vi "Go.vi"(9 "Timing Data":T1(array[cluster]), 10 "Control In":T2={"I-O.lvclass"=refnum, "Gantry"=refnum, "Dispenser"="COM1"}, 11 "Sensor Dispense in":refnum<class "Sensor Dispense.lvclass">) -> (2 "Control Out":T2={"I-O.lvclass"=refnum, "Gantry"=refnum, "Dispenser"="COM1"}, 3 "Sensor Dispense out":refnum<class "Sensor Dispense.lvclass">)   [LabVIEW 2018, in "Sensor Dispense.lvclass"]
uses:
  Sensor Dispense.lvclass
  C:/Users/HEP/Documents/GitHub/New folder/C/Users/HEP/Documents/GitHub/UCSB-Gantry-HEP-2018/Classes/Routine/Dispense/Dispense.lvclass
  Classes/Controller/Controllers.ctl
  Classes/Controller/I-O/I-O.lvclass
  C:/Program Files (x86)/Aerotech/A3200/LabVIEW/2010/Bin/Aerotech.A3200.dll
  Program Files (x86)/Aerotech/A3200/LabVIEW/2010/Bin/Aerotech.A3200.dll
  Sensor Dispense.lvclass/Sensor Dispense.ctl
  Classes/Controller/Motion/Motion.lvclass
  Classes/Controller/Dispenser/Dispenser.lvclass
  Classes/Controller/Motion/A3200/A3200.lvclass
  Classes/Controller/Controller.lvclass
panel:
  out "error out":errorcluster
  in  "error in (no error)":errorcluster
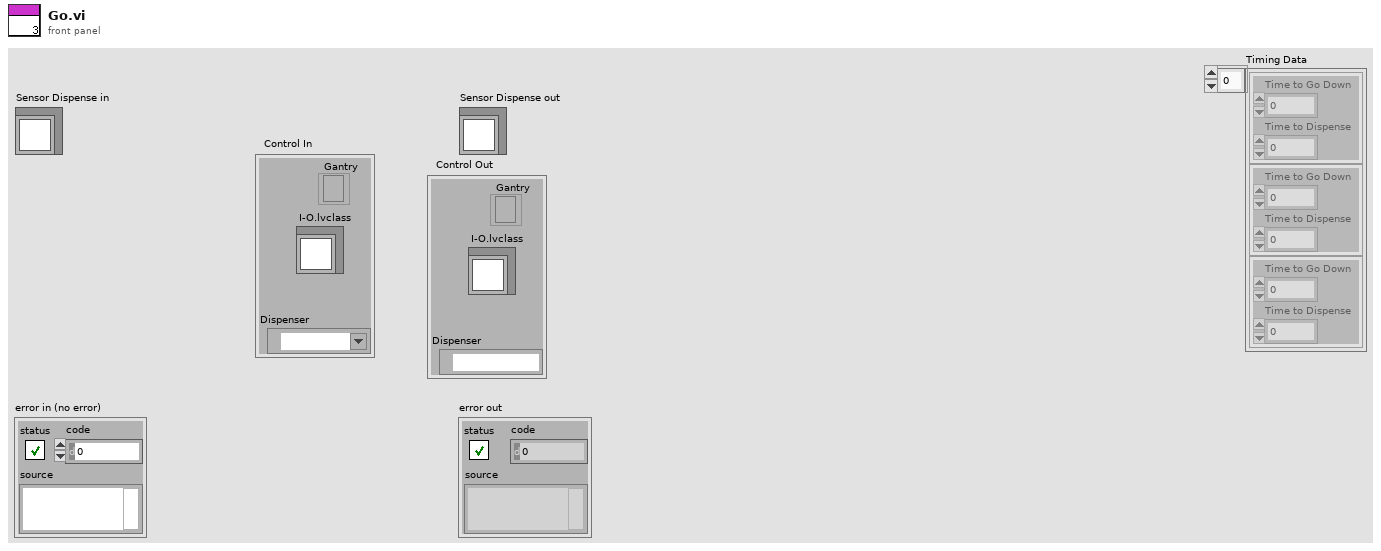
[diagram p1: front panel]
types:
  T1 = cluster{"Time to Go Down":i32, "Time to Dispense":i32}[]
  T2 = typedef "Controller.lvclass/Controllers.ctl" = cluster{"I-O.lvclass":refnum<class "I-O.lvclass">, "Gantry":refnum<k24>, "Dispenser":refnum<visa-resource-name>}
  T3 = cluster{"Endpoints":dbl[][], "Center":dbl[], "CW/CCW":dbl, "Dispense Type":enum16{"N-gon", "Square", "Arc", "Dot", "Line", "Circle"}}[]
  T4 = enum16{"N-gon", "Square", "Arc", "Dot", "Line", "Circle"}
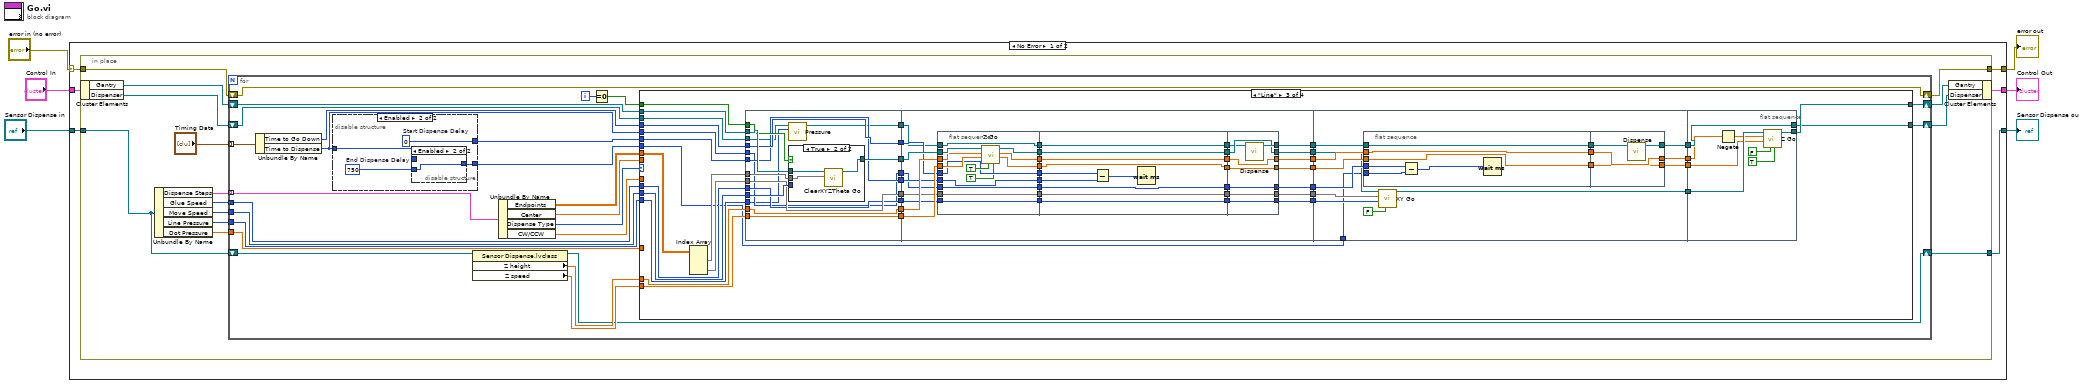
[diagram p0: block diagram]
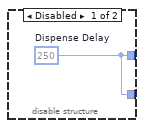
[diagram p2: hidden frame]
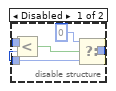
[diagram p3: hidden frame]
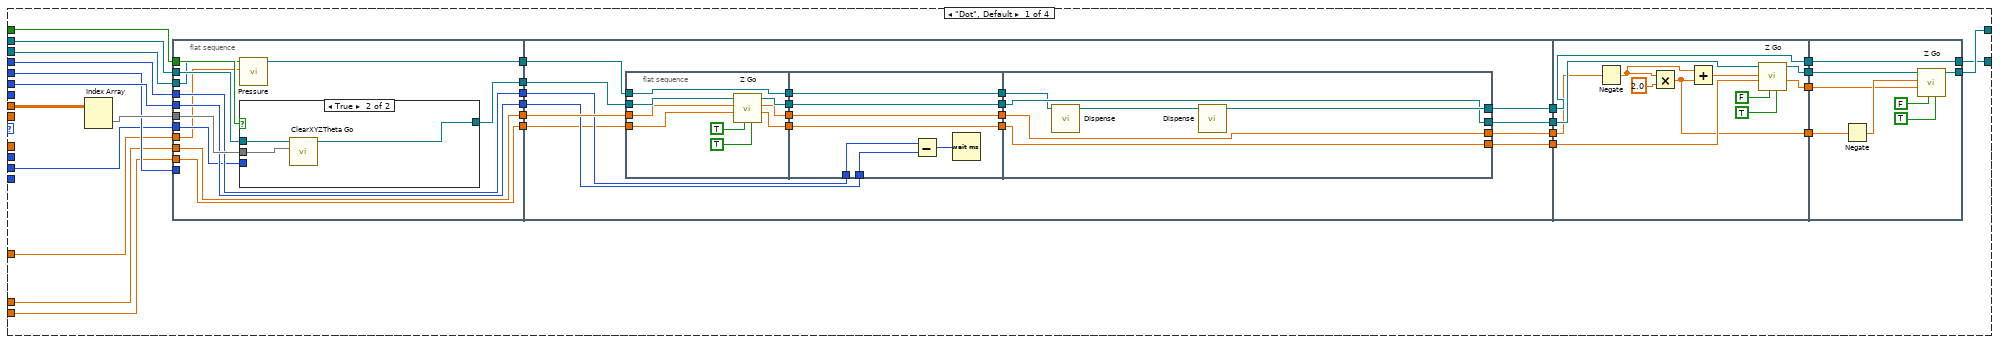
[diagram p4: hidden frame]
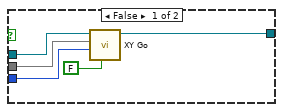
[diagram p5: hidden frame]
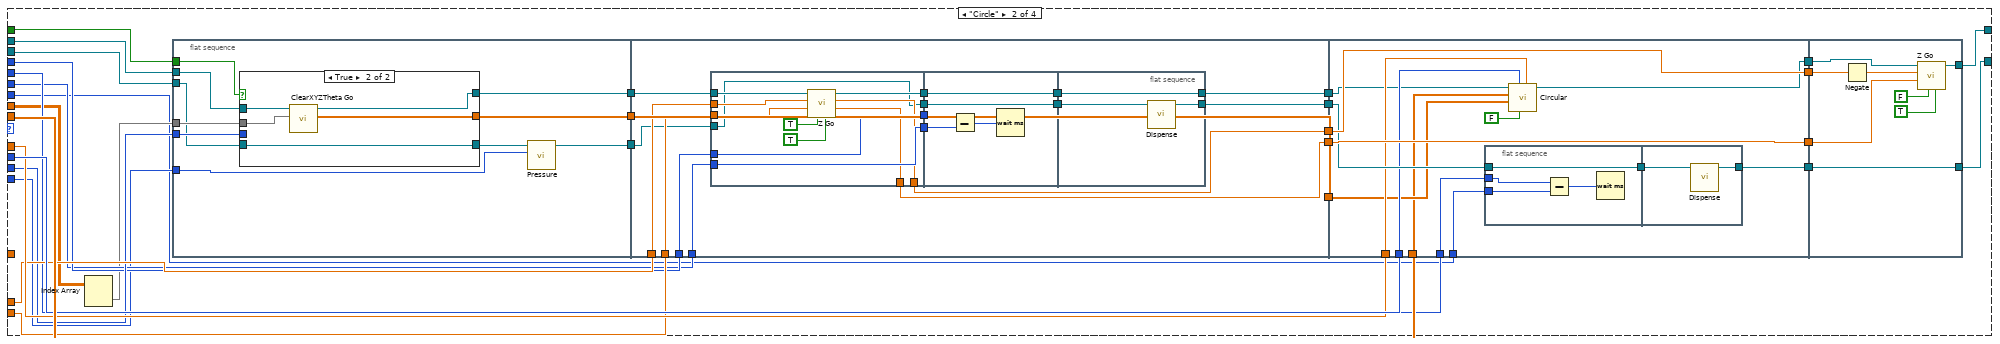
[diagram p6: hidden frame]
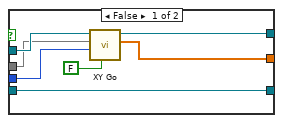
[diagram p7: hidden frame]
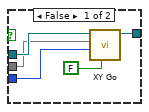
[diagram p8: hidden frame]
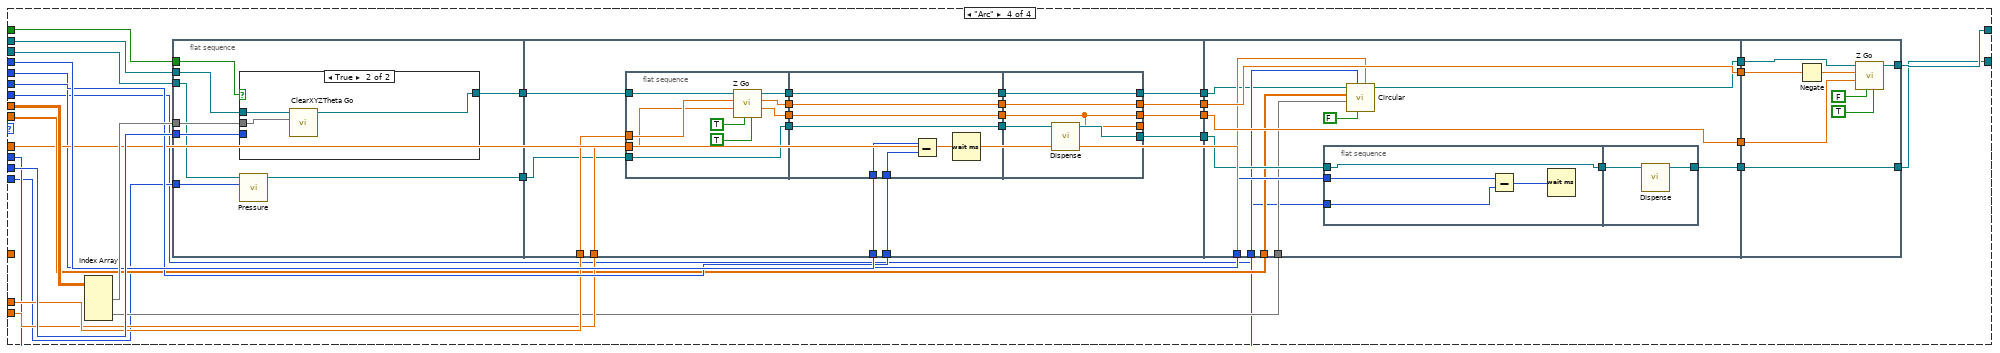
[diagram p9: hidden frame]
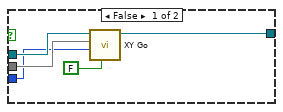
[diagram p10: hidden frame]
diagram:
  n1 = case shown="No Error" "error in (no error)" {
    selector: "error in (no error)" -> [w7 w559]
    tunnel: "Sensor Dispense in" -> [w12 w558]
    tunnel: [w11 w558] -> w5
    tunnel: "Control In" -> [w10 w557]
    tunnel: [w9 w557] -> w3
    tunnel: [w8 w559] -> w2
    frame No Error {
      n2 = in-place {
        in-place-border: w12 -> [w24]
        in-place-border: [w23] -> w11
        in-place-border: w7 -> [w17]
        in-place-border: [w16] -> w8
        n3 = in-place-cluster #1(w10) -> ("Gantry"=w25:refnum<k24>, "Dispenser"=w20:refnum<visa-resource-name>)
        n4 = Unbundle By Name(w24) -> ("Dispense Steps"=w21:T3, "Glue Speed"=w15:i32, "Move Speed"=w26:i32, "Line Pressure"=w13:i64, "Dot Pressure"=w14:dbl)
        n5 = for {
          tunnel: w26 -> [w51]
          shift-right: [w42] -> w22
          shift-left: w25 -> [w49]
          tunnel: w15 -> [w50]
          shift-right: [w34] -> w23
          shift-left: w24 -> [w47]
          tunnel: w21 -> [w44] mode=indexing
          shift-right: [w37] -> w18
          shift-left: w20 -> [w40]
          tunnel: "Timing Data" -> [w39] mode=indexing
          shift-right: [w29] -> w16
          shift-left: w17 -> [w29]
          tunnel: w14 -> [w31]
          tunnel: w13 -> [w30]
          i -> [w46]
          n6 = Unbundle By Name(w39) -> ("Time to Go Down"=w38:i32, "Time to Dispense"=w27:i32)
          n7 = disable-structure shown="Enabled" {
            disable-tunnel: [w52 w56] -> w33
            disable-tunnel: [w52 w54] -> w28
            disable-tunnel: w27 -> [_ w55]
            frame Disabled {
              w52 = 250  # Dispense Delay
            }
            frame Enabled {
              w53 = 750  # End Dispense Delay
              w56 = 0  # Start Dispense Delay
              n8 = disable-structure shown="Enabled" {
                disable-tunnel: w55 -> [w61 _]
                disable-tunnel: [w58 w62] -> w54
                disable-tunnel: w53 -> [w57 w62]
                frame Disabled {
                  n9 = Less?(x=w61, y=w57) -> (x < y?=w60:bool)
                  n10 = Select(t=0, s=w60, f=w57) -> (s? t:f=w58:i32)
                }
                frame Enabled {
                }
              }
            }
          }
          n11 = property class="Sensor Dispense.lvclass"(reference=w47) -> (reference out=w34:refnum<class "Sensor Dispense.lvclass">, "Z height"=w36:dbl, "Z speed"=w35:dbl)  [unwired: 1 in, 1 out]
          n12 = Unbundle By Name(w44) -> ("Endpoints"=w32:dbl[][], "Center"=w41:dbl[], "Dispense Type"=w43:T4, "CW/CCW"=w48:dbl)
          n13 = Equal To 0?(x=w46) -> (x = 0?=w45:bool)
          n14 = case shown="\"Line\"" w43 {
            tunnel: w41 -> [_ w196 _ w455]
            tunnel: w49 -> [w89 w197 w323 w464]
            tunnel: w51 -> [w72 w190 w322 w461]
            tunnel: [w88 w200 w319 w451] -> w42
            tunnel: w50 -> [_ w195 w309 w454]
            tunnel: w48 -> [_ w194 _ w453]
            tunnel: w35 -> [w80 w192 w306 w457]
            tunnel: w36 -> [w81 w193 w307 w458]
            tunnel: w45 -> [w90 w191 w321 w465]
            tunnel: w40 -> [w79 w174 w313 w447]
            tunnel: w38 -> [w77 w181 w311 w460]
            tunnel: w27 -> [w82 w182 w308 w452]
            tunnel: w33 -> [w83 w180 w312 w459]
            tunnel: [w87 w175 w316 w450] -> w37
            tunnel: w32 -> [w86 w179 w315 w463]
            tunnel: w31 -> [w71 _ _ _]
            tunnel: w30 -> [_ w172 w288 w446]
            tunnel: w28 -> [_ w171 w287 w445]
            frame "Dot", Default {
              n15 = Index Array(array=w86) -> (element=w85:dbl[])  [unwired: 2 in]
              n16 = flat-sequence {
                tunnel: w90 -> [w102]
                tunnel: w89 -> [w101]
                tunnel: w85 -> [w100]
                tunnel: [w99] -> w84
                tunnel: w83 -> [w96]
                tunnel: w82 -> [_]
                tunnel: w81 -> [w98]
                tunnel: w80 -> [w95]
                tunnel: w79 -> [w93]
                tunnel: [w98] -> w78
                tunnel: w77 -> [w97]
                tunnel: [w97] -> w76
                tunnel: [w96] -> w75
                tunnel: [w92] -> w74
                tunnel: [w95] -> w73
                tunnel: w72 -> [w94]
                tunnel: w71 -> [w91]
                tunnel: [w128] -> w68
                tunnel: w84 -> [w127]
                tunnel: [w124] -> w67
                tunnel: w78 -> [w123]
                tunnel: w76 -> [w122]
                tunnel: w75 -> [w121]
                tunnel: w74 -> [w120]
                tunnel: w73 -> [w117]
                tunnel: [w114] -> w66
                tunnel: [w113] -> w65
                tunnel: w68 -> [w161]
                tunnel: w67 -> [w160]
                tunnel: w66 -> [w159]
                tunnel: w65 -> [w156]
                tunnel: [w162] -> w70
                tunnel: [w161] -> w69
                tunnel: [w155] -> w64
                tunnel: [w151] -> w63
                tunnel: [w170] -> w87
                tunnel: [w168] -> w88
                tunnel: w70 -> [w169]
                tunnel: w69 -> [w170]
                tunnel: w64 -> [w166]
                tunnel: w63 -> [w163]
                frame #0 {
                  n17 = call "Pressure.vi"("Pressure"=w91, "VISA resource name"=w93) -> ("VISA resource name out"=w92:refnum<visa-resource-name>)  [unwired: 8 in, 1 out]
                  n18 = case shown="True" w102 {
                    tunnel: w101 -> [w107 w110]
                    tunnel: [w106 w109] -> w99
                    tunnel: w100 -> [w105 w108]
                    tunnel: w94 -> [w104 _]
                    frame False {
                      n19 = call "XY Go.vi"("return immediately"=FALSE, "Speed"=w104, "XY In"=w105, "Gantry In"=w107) -> ("Gantry Out"=w106:refnum<k24>)  [unwired: 5 in, 2 out]
                    }
                    frame True {
                      n20 = call "ClearXYZTheta Go.vi"("XYZTheta In"=w108, "Gantry In"=w110) -> ("Gantry Out"=w109:refnum<k24>)  [unwired: 7 in, 2 out]
                    }
                  }
                }
                frame #1 {
                  n21 = flat-sequence {
                    tunnel: w127 -> [w137]
                    tunnel: [w136] -> w125
                    tunnel: w123 -> [w129]
                    tunnel: w120 -> [w134]
                    tunnel: [w134] -> w119
                    tunnel: w117 -> [w133]
                    tunnel: [w132] -> w116
                    tunnel: [w131] -> w111
                    tunnel: [w144] -> w126
                    tunnel: w125 -> [w144]
                    tunnel: w122 -> [w143]
                    tunnel: w121 -> [w139]
                    tunnel: w119 -> [w142]
                    tunnel: [w142] -> w118
                    tunnel: w116 -> [w141]
                    tunnel: [w141] -> w115
                    tunnel: [w140] -> w112
                    tunnel: w111 -> [w140]
                    tunnel: [w150] -> w128
                    tunnel: w126 -> [w149]
                    tunnel: [w149] -> w124
                    tunnel: w118 -> [w148]
                    tunnel: w115 -> [w146]
                    tunnel: [w146] -> w114
                    tunnel: [w145] -> w113
                    tunnel: w112 -> [w145]
                    frame #0 {
                      n22 = call "Z Go.vi"("Increment"=TRUE, "Return Immediately"=TRUE, "Speed In"=w133, "Position In"=w129, "Gantry In"=w137) -> ("Speed Out"=w131:dbl, "Position Out"=w132:dbl, "Gantry Out"=w136:refnum<k24>)  [unwired: 3 in, 1 out]
                    }
                    frame #1 {
                      n23 = Subtract(x=w143, y=w139) -> (x-y=w138:i32)
                      n24 = Wait (ms)(milliseconds to wait=w138) -> ()  [unwired: 1 out]
                    }
                    frame #2 {
                      n25 = call "Dispense.vi"("Dispenser In"=w148) -> ("Dispenser Out"=w147:refnum<visa-resource-name>)  [unwired: 9 in, 1 out]
                      n26 = call "Dispense.vi"("Dispenser In"=w147) -> ("Dispenser Out"=w150:refnum<visa-resource-name>)  [unwired: 9 in, 1 out]
                    }
                  }
                }
                frame #2 {
                  n27 = Negate(x=w159) -> (-x=w153:dbl)
                  n28 = Multiply(x=w153, y=2.0) -> (x*y=w151:dbl)
                  n29 = Add(x=w153, y=w151) -> (x+y=w154:dbl)
                  n30 = call "Z Go.vi"("Increment"=TRUE, "Return Immediately"=FALSE, "Speed In"=w156, "Position In"=w154, "Gantry In"=w160) -> ("Speed Out"=w155:dbl, "Gantry Out"=w162:refnum<k24>)  [unwired: 3 in, 2 out]
                }
                frame #3 {
                  n31 = Negate(x=w163) -> (-x=w167:dbl)
                  n32 = call "Z Go.vi"("Increment"=TRUE, "Return Immediately"=FALSE, "Speed In"=w166, "Position In"=w167, "Gantry In"=w169) -> ("Gantry Out"=w168:refnum<k24>)  [unwired: 3 in, 3 out]
                }
              }
            }
            frame "Circle" {
              n33 = Index Array(array=w179) -> (element=w178:dbl[])  [unwired: 2 in]
              n34 = flat-sequence {
                tunnel: [w208] -> w199
                tunnel: w197 -> [w209]
                tunnel: w191 -> [w210]
                tunnel: w190 -> [w207]
                tunnel: [w206] -> w188
                tunnel: w178 -> [w205]
                tunnel: w174 -> [w204]
                tunnel: [w202] -> w173
                tunnel: w172 -> [w201]
                tunnel: w193 -> [w232]
                tunnel: w192 -> [w233]
                tunnel: [w239] -> w189
                tunnel: [w230] -> w187
                tunnel: [w231] -> w186
                tunnel: w188 -> [w239]
                tunnel: w199 -> [w229]
                tunnel: [w238] -> w183
                tunnel: w181 -> [w237]
                tunnel: w180 -> [w236]
                tunnel: [w226] -> w177
                tunnel: w173 -> [w225]
                tunnel: [w260] -> w198
                tunnel: [w272] -> w185
                tunnel: [w271] -> w184
                tunnel: w182 -> [w270]
                tunnel: w183 -> [w268]
                tunnel: w189 -> [w263]
                tunnel: w187 -> [w272]
                tunnel: w186 -> [w271]
                tunnel: w194 -> [w266]
                tunnel: w195 -> [w264]
                tunnel: w196 -> [w262]
                tunnel: w177 -> [w261]
                tunnel: [w269] -> w176
                tunnel: w171 -> [w259]
                tunnel: [w284] -> w200
                tunnel: w198 -> [w285]
                tunnel: w185 -> [w286]
                tunnel: w184 -> [w283]
                tunnel: w176 -> [w282]
                tunnel: [w282] -> w175
                frame #0 {
                  n35 = case shown="True" w210 {
                    tunnel: w209 -> [w217 w222]
                    tunnel: [w216 w221] -> w208
                    tunnel: w207 -> [w215 _]
                    tunnel: [w214 w219] -> w206
                    tunnel: w205 -> [w213 w220]
                    tunnel: w204 -> [w212 w218]
                    tunnel: [w212 w218] -> w203
                    frame False {
                      n36 = call "XY Go.vi"("return immediately"=FALSE, "Speed"=w215, "XY In"=w213, "Gantry In"=w217) -> ("XY Out"=w214:dbl[], "Gantry Out"=w216:refnum<k24>)  [unwired: 5 in, 1 out]
                    }
                    frame True {
                      n37 = call "ClearXYZTheta Go.vi"("XYZTheta In"=w220, "Gantry In"=w222) -> ("XYZTheta Out"=w219:dbl[], "Gantry Out"=w221:refnum<k24>)  [unwired: 7 in, 1 out]
                    }
                  }
                  n38 = call "Pressure.vi"("Pressure"=w201, "VISA resource name"=w203) -> ("VISA resource name out"=w202:refnum<visa-resource-name>)  [unwired: 8 in, 1 out]
                }
                frame #1 {
                  n39 = flat-sequence {
                    tunnel: w236 -> [w249]
                    tunnel: w237 -> [w250]
                    tunnel: [w250] -> w235
                    tunnel: [w249] -> w234
                    tunnel: w233 -> [w248]
                    tunnel: w232 -> [w247]
                    tunnel: [w246] -> w231
                    tunnel: [w245] -> w230
                    tunnel: w229 -> [w244]
                    tunnel: [w243] -> w228
                    tunnel: w225 -> [w241]
                    tunnel: [w241] -> w224
                    tunnel: w235 -> [w255]
                    tunnel: w234 -> [w254]
                    tunnel: w228 -> [w253]
                    tunnel: [w253] -> w227
                    tunnel: w224 -> [w252]
                    tunnel: [w252] -> w223
                    tunnel: [w258] -> w238
                    tunnel: w227 -> [w257]
                    tunnel: [w257] -> w226
                    tunnel: w223 -> [w256]
                    frame #0 {
                      n40 = call "Z Go.vi"("Increment"=TRUE, "Return Immediately"=TRUE ("return immediately"), "Speed In"=w248, "Position In"=w247, "Gantry In"=w244) -> ("Speed Out"=w246:dbl, "Position Out"=w245:dbl, "Gantry Out"=w243:refnum<k24>)  [unwired: 3 in, 1 out]
                    }
                    frame #1 {
                      n41 = Subtract(x=w255, y=w254) -> (x-y=w251:i32)
                      n42 = Wait (ms)(milliseconds to wait=w251) -> ()  [unwired: 1 out]
                    }
                    frame #2 {
                      n43 = call "Dispense.vi"("Dispenser In"=w256) -> ("Dispenser Out"=w258:refnum<visa-resource-name>)  [unwired: 9 in, 1 out]
                    }
                  }
                }
                frame #2 {
                  n44 = flat-sequence {
                    tunnel: [w274] -> w267
                    tunnel: w270 -> [w276]
                    tunnel: w268 -> [w274]
                    tunnel: w259 -> [w273]
                    tunnel: [w278] -> w269
                    tunnel: w267 -> [w277]
                    frame #0 {
                      n45 = Subtract(x=w276, y=w273) -> (x-y=w275:i32)
                      n46 = Wait (ms)(milliseconds to wait=w275) -> ()  [unwired: 1 out]
                    }
                    frame #1 {
                      n47 = call "Dispense.vi"("Dispenser In"=w277) -> ("Dispenser Out"=w278:refnum<visa-resource-name>)  [unwired: 9 in, 1 out]
                    }
                  }
                  n48 = call "Circular.vi"("Direction"=w266, "return immediately"=FALSE, "Speed"=w264, "XY End"=w263, "XY Center"=w262, "Gantry In"=w261) -> ("Gantry Out"=w260:refnum<k24>)  [unwired: 4 in, 1 out]
                }
                frame #3 {
                  n49 = Negate(x=w286) -> (-x=w281:dbl)
                  n50 = call "Z Go.vi"("Increment"=TRUE, "Return Immediately"=FALSE, "Speed In"=w283, "Position In"=w281, "Gantry In"=w285) -> ("Gantry Out"=w284:refnum<k24>)  [unwired: 3 in, 3 out]
                }
              }
            }
            frame "Line" {
              n51 = Index Array(array=w315) -> (element #1=w314:dbl[], element #2=w310:dbl[])  [unwired: 4 in]
              n52 = flat-sequence {
                tunnel: w323 -> [w338]
                tunnel: w322 -> [w337]
                tunnel: w321 -> [w336]
                tunnel: [w335] -> w320
                tunnel: w314 -> [w334]
                tunnel: w313 -> [w326]
                tunnel: w312 -> [w330]
                tunnel: w311 -> [w331]
                tunnel: w310 -> [w329]
                tunnel: w309 -> [w328]
                tunnel: w308 -> [w327]
                tunnel: w307 -> [w333]
                tunnel: w306 -> [w332]
                tunnel: [w333] -> w305
                tunnel: [w332] -> w304
                tunnel: [w331] -> w302
                tunnel: [w330] -> w301
                tunnel: [w325] -> w300
                tunnel: [w329] -> w298
                tunnel: [w328] -> w296
                tunnel: [w327] -> w294
                tunnel: w288 -> [w324]
                tunnel: w320 -> [w377]
                tunnel: [w378] -> w318
                tunnel: w305 -> [w376]
                tunnel: w304 -> [w375]
                tunnel: [w372] -> w303
                tunnel: w302 -> [w370]
                tunnel: w301 -> [w368]
                tunnel: w300 -> [w365]
                tunnel: [w364] -> w299
                tunnel: w298 -> [w361]
                tunnel: [w360] -> w297
                tunnel: w296 -> [w357]
                tunnel: [w353] -> w295
                tunnel: w294 -> [w354]
                tunnel: [w352] -> w291
                tunnel: [w349] -> w289
                tunnel: w318 -> [w424]
                tunnel: [w426] -> w317
                tunnel: w303 -> [w413]
                tunnel: w299 -> [w414]
                tunnel: w297 -> [w415]
                tunnel: w295 -> [w423]
                tunnel: [w412] -> w293
                tunnel: [w422] -> w292
                tunnel: w291 -> [w420]
                tunnel: [w419] -> w290
                tunnel: w289 -> [w417]
                tunnel: w287 -> [w411]
                tunnel: [w444] -> w319
                tunnel: w317 -> [w443]
                tunnel: [w443] -> w316
                tunnel: w293 -> [w442]
                tunnel: w292 -> [w441]
                tunnel: w290 -> [w439]
                frame #0 {
                  n53 = call "Pressure.vi"("Pressure"=w324, "VISA resource name"=w326) -> ("VISA resource name out"=w325:refnum<visa-resource-name>)  [unwired: 8 in, 1 out]
                  n54 = case shown="True" w336 {
                    tunnel: w338 -> [w343 w346]
                    tunnel: w337 -> [w342 _]
                    tunnel: [w341 w345] -> w335
                    tunnel: w334 -> [w340 w344]
                    frame False {
                      n55 = call "XY Go.vi"("return immediately"=FALSE, "Speed"=w342, "XY In"=w340, "Gantry In"=w343) -> ("Gantry Out"=w341:refnum<k24>)  [unwired: 5 in, 2 out]
                    }
                    frame True {
                      n56 = call "ClearXYZTheta Go.vi"("XYZTheta In"=w344, "Gantry In"=w346) -> ("Gantry Out"=w345:refnum<k24>)  [unwired: 7 in, 2 out]
                    }
                  }
                }
                frame #1 {
                  n57 = flat-sequence {
                    tunnel: w377 -> [w392]
                    tunnel: w376 -> [w391]
                    tunnel: w375 -> [w390]
                    tunnel: [w388] -> w374
                    tunnel: [w387] -> w371
                    tunnel: w370 -> [w387]
                    tunnel: [w386] -> w369
                    tunnel: w368 -> [w386]
                    tunnel: [w385] -> w366
                    tunnel: w365 -> [w385]
                    tunnel: [w384] -> w362
                    tunnel: w361 -> [w384]
                    tunnel: [w383] -> w358
                    tunnel: w357 -> [w383]
                    tunnel: [w382] -> w355
                    tunnel: w354 -> [w382]
                    tunnel: [w381] -> w350
                    tunnel: [w380] -> w347
                    tunnel: w374 -> [w402]
                    tunnel: [w402] -> w373
                    tunnel: w371 -> [w401]
                    tunnel: w369 -> [w396]
                    tunnel: [w400] -> w367
                    tunnel: w366 -> [w400]
                    tunnel: [w399] -> w363
                    tunnel: w362 -> [w399]
                    tunnel: [w398] -> w359
                    tunnel: w358 -> [w398]
                    tunnel: [w397] -> w356
                    tunnel: w355 -> [w397]
                    tunnel: [w395] -> w351
                    tunnel: w350 -> [w395]
                    tunnel: [w394] -> w348
                    tunnel: w347 -> [w394]
                    tunnel: [w410] -> w378
                    tunnel: w373 -> [w409]
                    tunnel: [w409] -> w372
                    tunnel: w367 -> [w405]
                    tunnel: [w408] -> w364
                    tunnel: w363 -> [w408]
                    tunnel: [w407] -> w360
                    tunnel: w359 -> [w407]
                    tunnel: w356 -> [w406]
                    tunnel: [w406] -> w353
                    tunnel: [w404] -> w352
                    tunnel: w351 -> [w404]
                    tunnel: [w403] -> w349
                    tunnel: w348 -> [w403]
                    frame #0 {
                      n58 = call "Z Go.vi"("Increment"=TRUE, "Return Immediately"=TRUE, "Speed In"=w390, "Position In"=w391, "Gantry In"=w392) -> ("Speed Out"=w380:dbl, "Position Out"=w381:dbl, "Gantry Out"=w388:refnum<k24>)  [unwired: 3 in, 1 out]
                    }
                    frame #1 {
                      n59 = Subtract(x=w401, y=w396) -> (x-y=w393:i32)
                      n60 = Wait (ms)(milliseconds to wait=w393) -> ()  [unwired: 1 out]
                    }
                    frame #2 {
                      n61 = call "Dispense.vi"("Dispenser In"=w405) -> ("Dispenser Out"=w410:refnum<visa-resource-name>)  [unwired: 9 in, 1 out]
                    }
                  }
                }
                frame #2 {
                  n62 = flat-sequence {
                    tunnel: [w432] -> w425
                    tunnel: [w430] -> w421
                    tunnel: [w429] -> w418
                    tunnel: w424 -> [w432]
                    tunnel: w423 -> [w431]
                    tunnel: w420 -> [w430]
                    tunnel: w417 -> [w429]
                    tunnel: w411 -> [w427]
                    tunnel: [w436] -> w426
                    tunnel: w425 -> [w435]
                    tunnel: [w434] -> w422
                    tunnel: w421 -> [w434]
                    tunnel: [w433] -> w419
                    tunnel: w418 -> [w433]
                    frame #0 {
                      n63 = Subtract(x=w431, y=w427) -> (x-y=w428:i32)
                      n64 = Wait (ms)(milliseconds to wait=w428) -> ()  [unwired: 1 out]
                    }
                    frame #1 {
                      n65 = call "Dispense.vi"("Dispenser In"=w435) -> ("Dispenser Out"=w436:refnum<visa-resource-name>)  [unwired: 9 in, 1 out]
                    }
                  }
                  n66 = call "XY Go.vi"("return immediately"=FALSE, "Speed"=w415, "XY In"=w414, "Gantry In"=w413) -> ("Gantry Out"=w412:refnum<k24>)  [unwired: 5 in, 2 out]
                }
                frame #3 {
                  n67 = Negate(x=w441) -> (-x=w440:dbl)
                  n68 = call "Z Go.vi"("Increment"=TRUE, "Return Immediately"=FALSE, "Speed In"=w439, "Position In"=w440, "Gantry In"=w442) -> ("Gantry Out"=w444:refnum<k24>)  [unwired: 3 in, 3 out]
                }
              }
            }
            frame "Arc" {
              n69 = Index Array(array=w463) -> (element #1=w462:dbl[], element #2=w456:dbl[])  [unwired: 4 in]
              n70 = flat-sequence {
                tunnel: [w481] -> w473
                tunnel: w465 -> [w480]
                tunnel: w464 -> [w479]
                tunnel: w462 -> [w478]
                tunnel: w461 -> [w477]
                tunnel: [w476] -> w448
                tunnel: w447 -> [w475]
                tunnel: w446 -> [w474]
                tunnel: w473 -> [w506]
                tunnel: [w507] -> w472
                tunnel: [w503] -> w471
                tunnel: [w500] -> w470
                tunnel: [w497] -> w469
                tunnel: w460 -> [w496]
                tunnel: w459 -> [w495]
                tunnel: w458 -> [w494]
                tunnel: w457 -> [w493]
                tunnel: w448 -> [w492]
                tunnel: w472 -> [w538]
                tunnel: [w539] -> w468
                tunnel: w471 -> [w531]
                tunnel: w470 -> [w542]
                tunnel: [w542] -> w467
                tunnel: w469 -> [w541]
                tunnel: [w541] -> w466
                tunnel: w456 -> [w533]
                tunnel: w455 -> [w532]
                tunnel: w454 -> [w534]
                tunnel: w453 -> [w536]
                tunnel: w452 -> [w540]
                tunnel: [w530] -> w449
                tunnel: w445 -> [w529]
                tunnel: [w556] -> w451
                tunnel: w468 -> [w555]
                tunnel: [w555] -> w450
                tunnel: w467 -> [w553]
                tunnel: w466 -> [w551]
                tunnel: w449 -> [w554]
                frame #0 {
                  n71 = case shown="True" w480 {
                    tunnel: [w486 w489] -> w481
                    tunnel: w479 -> [w485 w488]
                    tunnel: w478 -> [w484 w487]
                    tunnel: w477 -> [w483 _]
                    frame False {
                      n72 = call "XY Go.vi"("return immediately"=FALSE, "Speed"=w483, "XY In"=w484, "Gantry In"=w485) -> ("Gantry Out"=w486:refnum<k24>)  [unwired: 5 in, 2 out]
                    }
                    frame True {
                      n73 = call "ClearXYZTheta Go.vi"("XYZTheta In"=w487, "Gantry In"=w488) -> ("Gantry Out"=w489:refnum<k24>)  [unwired: 7 in, 2 out]
                    }
                  }
                  n74 = call "Pressure.vi"("Pressure"=w474, "VISA resource name"=w475) -> ("VISA resource name out"=w476:refnum<visa-resource-name>)  [unwired: 8 in, 1 out]
                }
                frame #1 {
                  n75 = flat-sequence {
                    tunnel: w506 -> [w516]
                    tunnel: [w514] -> w505
                    tunnel: [w513] -> w502
                    tunnel: [w512] -> w501
                    tunnel: w494 -> [w511]
                    tunnel: w493 -> [w510]
                    tunnel: w492 -> [w508]
                    tunnel: [w508] -> w491
                    tunnel: w505 -> [w523]
                    tunnel: [w523] -> w504
                    tunnel: w502 -> [w522]
                    tunnel: w501 -> [w521]
                    tunnel: [w522] -> w499
                    tunnel: [w521] -> w498
                    tunnel: w496 -> [w520]
                    tunnel: w495 -> [w519]
                    tunnel: w491 -> [w518]
                    tunnel: [w518] -> w490
                    tunnel: [w528] -> w507
                    tunnel: w504 -> [w527]
                    tunnel: [w527] -> w503
                    tunnel: [w526] -> w500
                    tunnel: w499 -> [w526]
                    tunnel: w498 -> [w525]
                    tunnel: [w525] -> _
                    tunnel: [w525] -> w497
                    tunnel: w490 -> [w524]
                    frame #0 {
                      n76 = call "Z Go.vi"("Increment"=TRUE, "Return Immediately"=TRUE, "Speed In"=w510, "Position In"=w511, "Gantry In"=w516) -> ("Speed Out"=w512:dbl, "Position Out"=w513:dbl, "Gantry Out"=w514:refnum<k24>)  [unwired: 3 in, 1 out]
                    }
                    frame #1 {
                      n77 = Subtract(x=w520, y=w519) -> (x-y=w517:i32)
                      n78 = Wait (ms)(milliseconds to wait=w517) -> ()  [unwired: 1 out]
                    }
                    frame #2 {
                      n79 = call "Dispense.vi"("Dispenser In"=w524) -> ("Dispenser Out"=w528:refnum<visa-resource-name>)  [unwired: 9 in, 1 out]
                    }
                  }
                }
                frame #2 {
                  n80 = flat-sequence {
                    tunnel: [w544] -> w537
                    tunnel: w540 -> [w546]
                    tunnel: w538 -> [w544]
                    tunnel: w529 -> [w543]
                    tunnel: [w548] -> w539
                    tunnel: w537 -> [w547]
                    frame #0 {
                      n81 = Subtract(x=w546, y=w543) -> (x-y=w545:i32)
                      n82 = Wait (ms)(milliseconds to wait=w545) -> ()  [unwired: 1 out]
                    }
                    frame #1 {
                      n83 = call "Dispense.vi"("Dispenser In"=w547) -> ("Dispenser Out"=w548:refnum<visa-resource-name>)  [unwired: 9 in, 1 out]
                    }
                  }
                  n84 = call "Circular.vi"("Direction"=w536, "return immediately"=FALSE, "Speed"=w534, "XY End"=w533, "XY Center"=w532, "Gantry In"=w531) -> ("Gantry Out"=w530:refnum<k24>)  [unwired: 4 in, 1 out]
                }
                frame #3 {
                  n85 = Negate(x=w553) -> (-x=w552:dbl)
                  n86 = call "Z Go.vi"("Increment"=TRUE, "Return Immediately"=FALSE, "Speed In"=w551, "Position In"=w552, "Gantry In"=w554) -> ("Gantry Out"=w556:refnum<k24>)  [unwired: 3 in, 3 out]
                }
              }
            }
          }
        }
        n87 = in-place-cluster #1("Gantry"=w22, "Dispenser"=w18) -> (w9:T2)
      }
    }
    frame Error {
    }
  }
  "error out" <- w2
  "Sensor Dispense out" <- w5
  "Control Out" <- w3
